vi "IsTokenEqual.vi"(8 "error in (no error)":errorcluster, 10 "EventToken":refnum<class "EventToken.lvclass">, 11 "EventToken in":refnum<class "EventToken.lvclass">) -> (0 "error out":errorcluster, 1 "Is Equal?":bool, 2 "EventToken":refnum<class "EventToken.lvclass">, 3 "EventToken out":refnum<class "EventToken.lvclass">)   [LabVIEW 2009, in "EventManagerLibrary.lvlib" / "EventToken.lvclass"]
doc: "Returns TRUE if two tokens are identical. Tokens may refer to the same event and not be identical."
uses:
  EventToken.lvclass
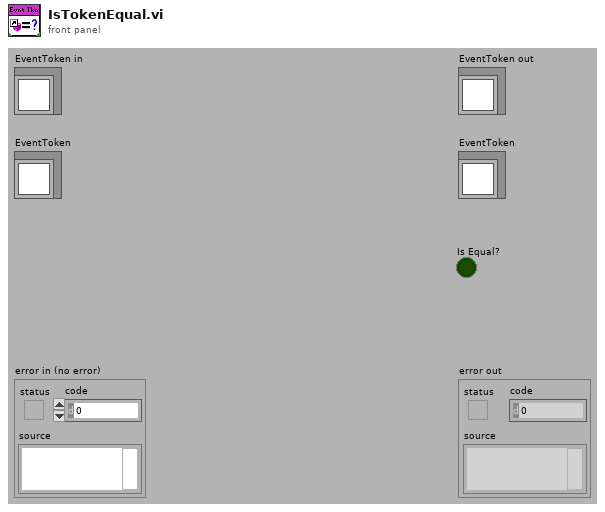
[diagram p1: front panel]
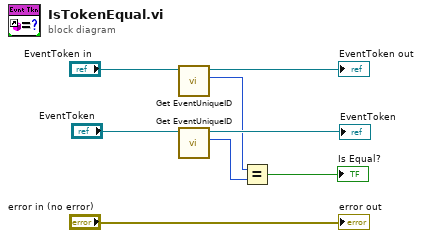
[diagram p0: block diagram]
diagram:
  n1 = call "Get EventUniqueID.vi"("EventToken in"="EventToken in") -> ("EventRefnum"=w2:i32, "EventToken out"=→"EventToken out":refnum<class "EventToken.lvclass">)  [unwired: 8 in, 1 out]
  n2 = call "Get EventUniqueID.vi"("EventToken in"="EventToken") -> ("EventRefnum"=w1:i32, "EventToken out"=→"EventToken":refnum<class "EventToken.lvclass">)  [unwired: 8 in, 1 out]
  n3 = Equal?(x=w2, y=w1) -> (x = y?=→"Is Equal?":bool)
  "error out" <- "error in (no error)"
